vi "set decimali misure.vi"(6 "medie":i32[](array[numeric]), 8 "Abilita medie":bool, 9 "Filtro":bool[](array[boolean]), 10 "MISURE in":string[](array[string]), 11 "decimali":i32[](array[numeric])) -> (3 "MISURE out":string[](array[string]))   [LabVIEW 2019]
uses:
  <vilib>/ptbypt/NI_PtbyPt.lvlib
panel:
  out "Array":i32[](array[numeric])
  out "Numeric":i32
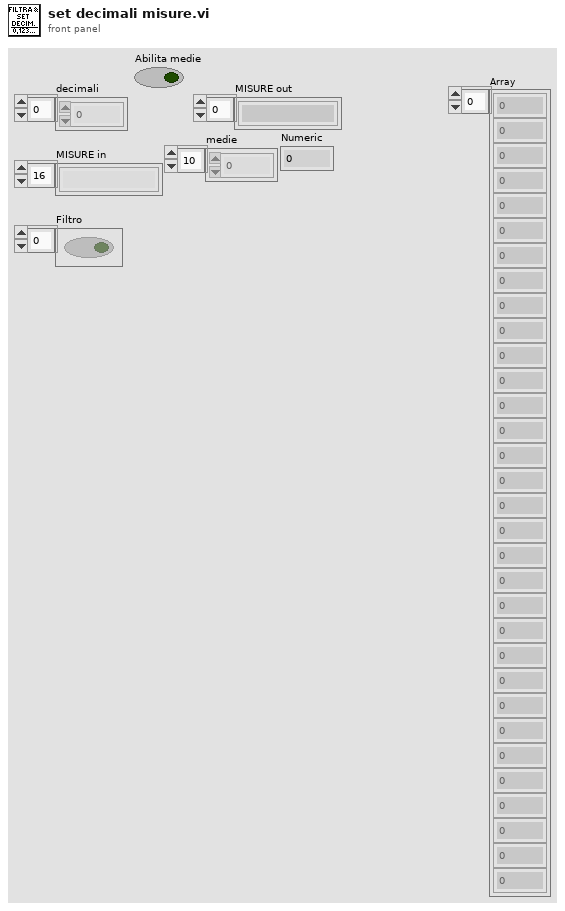
[diagram p1: front panel]
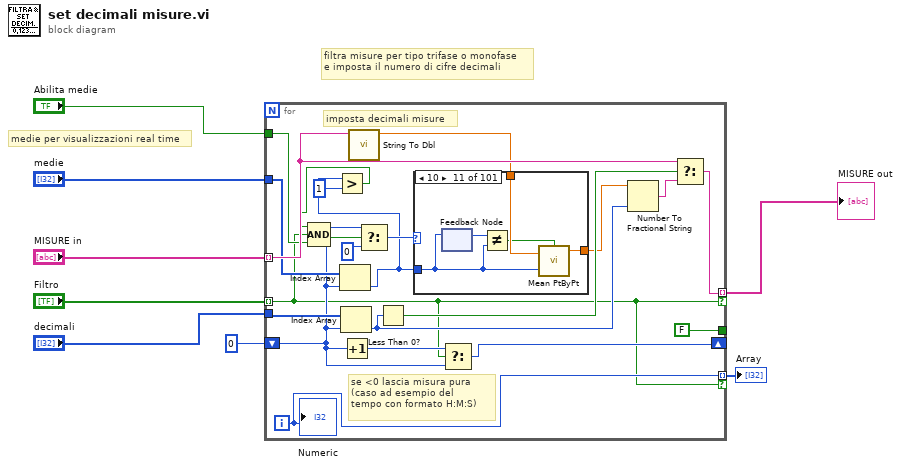
[diagram p0: block diagram]
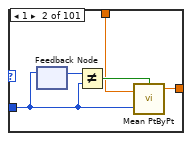
[diagram p3: hidden frame]
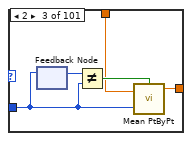
[diagram p4: hidden frame]
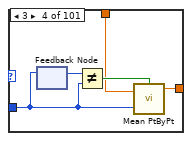
[diagram p5: hidden frame]
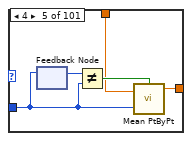
[diagram p6: hidden frame]
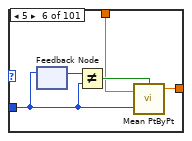
[diagram p7: hidden frame]
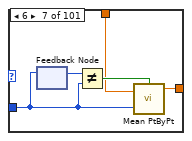
[diagram p8: hidden frame]
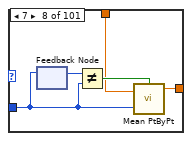
[diagram p9: hidden frame]
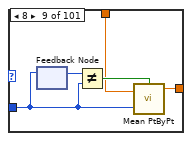
[diagram p10: hidden frame]
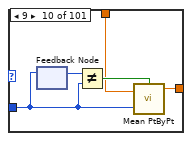
[diagram p11: hidden frame]
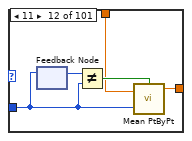
[diagram p12: hidden frame]
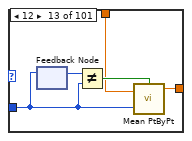
[diagram p13: hidden frame]
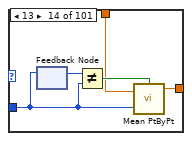
[diagram p14: hidden frame]
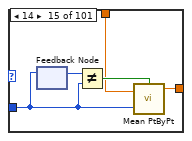
[diagram p15: hidden frame]
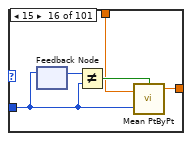
[diagram p16: hidden frame]
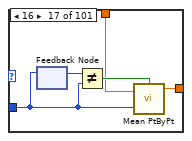
[diagram p17: hidden frame]
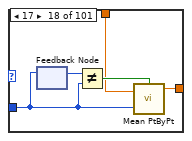
[diagram p18: hidden frame]
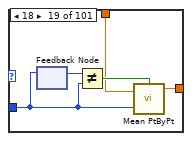
[diagram p19: hidden frame]
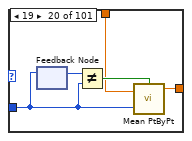
[diagram p20: hidden frame]
diagram:
  # "medie per visualizzazioni real time"
  # "filtra misure per tipo trifase o monofase\ne imposta il numero di cifre decimali"
  n1 = for {
    tunnel: "MISURE in" -> [w23] mode=indexing
    tunnel: [w24] -> w8 mode=indexing if=w9
    tunnel: [FALSE] -> _
    shift-right: [w29] -> _
    shift-left: 0 -> [w16]
    tunnel: "Filtro" -> [w9] mode=indexing
    tunnel: "decimali" -> [w27]
    tunnel: "medie" -> [w17]
    tunnel: "Abilita medie" -> [w15]
    tunnel: [w10] -> w1 mode=indexing if=w9
    i -> [w10]
    # "se <0 lascia misura pura\n(caso ad esempio del\ntempo con formato H:M:S)"
    # "imposta decimali misure"
    n2 = Index Array(array=w17, index=w16) -> (element=w13:i32)
    n3 = Greater?(x=w13, y=1) -> (0:w11:bool)
    n4 = Compound Arithmetic op=AND(w11, w9, w15) -> (w14:bool)
    n5 = Index Array(array=w27, index=w16) -> (element=w26:i32)
    n6 = Increment(x=w16) -> (x+1=w28:i32)
    n7 = call "String To Dbl.vi"("String"=w23) -> ("Numeric"=w20:dbl)  [unwired: 10 in]
    n8 = Select(t=w16, s=w14, f=0) -> (s? t:f=w19:i32)
    n9 = Less Than 0?(x=w26) -> (x < 0?=w22:bool)
    n10 = case shown="10" w19 {
      tunnel: w13 -> [_ w32 w37 w42 w47 w52 w57 w62 w67 w72 w78 w82 w87 w92 w97 w102 w107 w112 w117 w122 w127 w132 w137 w142 w147 w152 w157 w162 w167 w172 w177 w182 w187 w192 w197 w202 w207 w212 w217 w222 w227 w232 w237 w242 w247 w252 w257 w262 w267 w272 w277 w282 w287 w292 w297 w302 w307 w312 w317 w322 w327 w332 w337 w342 w347 w352 w357 w362 w367 w372 w377 w382 w387 w392 w397 w402 w407 w412 w417 w422 w427 w432 w437 w442 w447 w452 w457 w462 w467 w472 w477 w482 w487 w492 w497 w502 w507 w512 w517 w522 w527]
      tunnel: [w31 w34 w39 w44 w49 w54 w59 w64 w69 w74 w80 w84 w89 w94 w99 w104 w109 w114 w119 w124 w129 w134 w139 w144 w149 w154 w159 w164 w169 w174 w179 w184 w189 w194 w199 w204 w209 w214 w219 w224 w229 w234 w239 w244 w249 w254 w259 w264 w269 w274 w279 w284 w289 w294 w299 w304 w309 w314 w319 w324 w329 w334 w339 w344 w349 w354 w359 w364 w369 w374 w379 w384 w389 w394 w399 w404 w409 w414 w419 w424 w429 w434 w439 w444 w449 w454 w459 w464 w469 w474 w479 w484 w489 w494 w499 w504 w509 w514 w519 w524 w529] -> w21
      tunnel: w20 -> [w31 w33 w38 w43 w48 w53 w58 w63 w68 w73 w79 w83 w88 w93 w98 w103 w108 w113 w118 w123 w128 w133 w138 w143 w148 w153 w158 w163 w168 w173 w178 w183 w188 w193 w198 w203 w208 w213 w218 w223 w228 w233 w238 w243 w248 w253 w258 w263 w268 w273 w278 w283 w288 w293 w298 w303 w308 w313 w318 w323 w328 w333 w338 w343 w348 w353 w358 w363 w368 w373 w378 w383 w388 w393 w398 w403 w408 w413 w418 w423 w428 w433 w438 w443 w448 w453 w458 w463 w468 w473 w478 w483 w488 w493 w498 w503 w508 w513 w518 w523 w528]
      frame 0, Default {
      }
      frame 1 {
        n11 = feedback #1() -> (w35:i32)  [unwired: 1 in]
        n12 = feedback-in #1(w32) -> ()
        n13 = Not Equal?(x=w35, y=w32) -> (x != y?=w36:bool)
        n14 = call <vilib>:"Mean PtByPt.vi"("x"=w33, "sample length"=w32, "initialize"=w36) -> ("mean"=w34:dbl)  [unwired: 1 in, 1 out]
      }
      frame 2 {
        n15 = feedback #2() -> (w40:i32)  [unwired: 1 in]
        n16 = feedback-in #2(w37) -> ()
        n17 = Not Equal?(x=w40, y=w37) -> (x != y?=w41:bool)
        n18 = call <vilib>:"Mean PtByPt.vi"("x"=w38, "sample length"=w37, "initialize"=w41) -> ("mean"=w39:dbl)  [unwired: 1 in, 1 out]
      }
      frame 3 {
        n19 = feedback #3() -> (w45:i32)  [unwired: 1 in]
        n20 = feedback-in #3(w42) -> ()
        n21 = Not Equal?(x=w45, y=w42) -> (x != y?=w46:bool)
        n22 = call <vilib>:"Mean PtByPt.vi"("x"=w43, "sample length"=w42, "initialize"=w46) -> ("mean"=w44:dbl)  [unwired: 1 in, 1 out]
      }
      frame 4 {
        n23 = feedback #4() -> (w50:i32)  [unwired: 1 in]
        n24 = feedback-in #4(w47) -> ()
        n25 = Not Equal?(x=w50, y=w47) -> (x != y?=w51:bool)
        n26 = call <vilib>:"Mean PtByPt.vi"("x"=w48, "sample length"=w47, "initialize"=w51) -> ("mean"=w49:dbl)  [unwired: 1 in, 1 out]
      }
      frame 5 {
        n27 = feedback #5() -> (w55:i32)  [unwired: 1 in]
        n28 = feedback-in #5(w52) -> ()
        n29 = Not Equal?(x=w55, y=w52) -> (x != y?=w56:bool)
        n30 = call <vilib>:"Mean PtByPt.vi"("x"=w53, "sample length"=w52, "initialize"=w56) -> ("mean"=w54:dbl)  [unwired: 1 in, 1 out]
      }
      frame 6 {
        n31 = feedback #6() -> (w60:i32)  [unwired: 1 in]
        n32 = feedback-in #6(w57) -> ()
        n33 = Not Equal?(x=w60, y=w57) -> (x != y?=w61:bool)
        n34 = call <vilib>:"Mean PtByPt.vi"("x"=w58, "sample length"=w57, "initialize"=w61) -> ("mean"=w59:dbl)  [unwired: 1 in, 1 out]
      }
      frame 7 {
        n35 = feedback #7() -> (w65:i32)  [unwired: 1 in]
        n36 = feedback-in #7(w62) -> ()
        n37 = Not Equal?(x=w65, y=w62) -> (x != y?=w66:bool)
        n38 = call <vilib>:"Mean PtByPt.vi"("x"=w63, "sample length"=w62, "initialize"=w66) -> ("mean"=w64:dbl)  [unwired: 1 in, 1 out]
      }
      frame 8 {
        n39 = feedback #8() -> (w70:i32)  [unwired: 1 in]
        n40 = feedback-in #8(w67) -> ()
        n41 = Not Equal?(x=w70, y=w67) -> (x != y?=w71:bool)
        n42 = call <vilib>:"Mean PtByPt.vi"("x"=w68, "sample length"=w67, "initialize"=w71) -> ("mean"=w69:dbl)  [unwired: 1 in, 1 out]
      }
      frame 9 {
        n43 = feedback #9() -> (w75:i32)  [unwired: 1 in]
        n44 = feedback-in #9(w72) -> ()
        n45 = Not Equal?(x=w75, y=w72) -> (x != y?=w76:bool)
        n46 = call <vilib>:"Mean PtByPt.vi"("x"=w73, "sample length"=w72, "initialize"=w76) -> ("mean"=w74:dbl)  [unwired: 1 in, 1 out]
      }
      frame 10 {
        n47 = feedback #10() -> (w81:i32)  [unwired: 1 in]
        n48 = feedback-in #10(w78) -> ()
        n49 = Not Equal?(x=w81, y=w78) -> (x != y?=w77:bool)
        n50 = call <vilib>:"Mean PtByPt.vi"("x"=w79, "sample length"=w78, "initialize"=w77) -> ("mean"=w80:dbl)  [unwired: 1 in, 1 out]
      }
      frame 11 {
        n51 = feedback #11() -> (w85:i32)  [unwired: 1 in]
        n52 = feedback-in #11(w82) -> ()
        n53 = Not Equal?(x=w85, y=w82) -> (x != y?=w86:bool)
        n54 = call <vilib>:"Mean PtByPt.vi"("x"=w83, "sample length"=w82, "initialize"=w86) -> ("mean"=w84:dbl)  [unwired: 1 in, 1 out]
      }
      frame 12 {
        n55 = feedback #12() -> (w90:i32)  [unwired: 1 in]
        n56 = feedback-in #12(w87) -> ()
        n57 = Not Equal?(x=w90, y=w87) -> (x != y?=w91:bool)
        n58 = call <vilib>:"Mean PtByPt.vi"("x"=w88, "sample length"=w87, "initialize"=w91) -> ("mean"=w89:dbl)  [unwired: 1 in, 1 out]
      }
      frame 13 {
        n59 = feedback #13() -> (w95:i32)  [unwired: 1 in]
        n60 = feedback-in #13(w92) -> ()
        n61 = Not Equal?(x=w95, y=w92) -> (x != y?=w96:bool)
        n62 = call <vilib>:"Mean PtByPt.vi"("x"=w93, "sample length"=w92, "initialize"=w96) -> ("mean"=w94:dbl)  [unwired: 1 in, 1 out]
      }
      frame 14 {
        n63 = feedback #14() -> (w100:i32)  [unwired: 1 in]
        n64 = feedback-in #14(w97) -> ()
        n65 = Not Equal?(x=w100, y=w97) -> (x != y?=w101:bool)
        n66 = call <vilib>:"Mean PtByPt.vi"("x"=w98, "sample length"=w97, "initialize"=w101) -> ("mean"=w99:dbl)  [unwired: 1 in, 1 out]
      }
      frame 15 {
        n67 = feedback #15() -> (w105:i32)  [unwired: 1 in]
        n68 = feedback-in #15(w102) -> ()
        n69 = Not Equal?(x=w105, y=w102) -> (x != y?=w106:bool)
        n70 = call <vilib>:"Mean PtByPt.vi"("x"=w103, "sample length"=w102, "initialize"=w106) -> ("mean"=w104:dbl)  [unwired: 1 in, 1 out]
      }
      frame 16 {
        n71 = feedback #16() -> (w110:i32)  [unwired: 1 in]
        n72 = feedback-in #16(w107) -> ()
        n73 = Not Equal?(x=w110, y=w107) -> (x != y?=w111:bool)
        n74 = call <vilib>:"Mean PtByPt.vi"("x"=w108, "sample length"=w107, "initialize"=w111) -> ("mean"=w109:dbl)  [unwired: 1 in, 1 out]
      }
      frame 17 {
        n75 = feedback #17() -> (w115:i32)  [unwired: 1 in]
        n76 = feedback-in #17(w112) -> ()
        n77 = Not Equal?(x=w115, y=w112) -> (x != y?=w116:bool)
        n78 = call <vilib>:"Mean PtByPt.vi"("x"=w113, "sample length"=w112, "initialize"=w116) -> ("mean"=w114:dbl)  [unwired: 1 in, 1 out]
      }
      frame 18 {
        n79 = feedback #18() -> (w120:i32)  [unwired: 1 in]
        n80 = feedback-in #18(w117) -> ()
        n81 = Not Equal?(x=w120, y=w117) -> (x != y?=w121:bool)
        n82 = call <vilib>:"Mean PtByPt.vi"("x"=w118, "sample length"=w117, "initialize"=w121) -> ("mean"=w119:dbl)  [unwired: 1 in, 1 out]
      }
      frame 19 {
        n83 = feedback #19() -> (w125:i32)  [unwired: 1 in]
        n84 = feedback-in #19(w122) -> ()
        n85 = Not Equal?(x=w125, y=w122) -> (x != y?=w126:bool)
        n86 = call <vilib>:"Mean PtByPt.vi"("x"=w123, "sample length"=w122, "initialize"=w126) -> ("mean"=w124:dbl)  [unwired: 1 in, 1 out]
      }
      frame 20 {
        n87 = feedback #20() -> (w130:i32)  [unwired: 1 in]
        n88 = feedback-in #20(w127) -> ()
        n89 = Not Equal?(x=w130, y=w127) -> (x != y?=w131:bool)
        n90 = call <vilib>:"Mean PtByPt.vi"("x"=w128, "sample length"=w127, "initialize"=w131) -> ("mean"=w129:dbl)  [unwired: 1 in, 1 out]
      }
      frame 21 {
        n91 = feedback #21() -> (w135:i32)  [unwired: 1 in]
        n92 = feedback-in #21(w132) -> ()
        n93 = Not Equal?(x=w135, y=w132) -> (x != y?=w136:bool)
        n94 = call <vilib>:"Mean PtByPt.vi"("x"=w133, "sample length"=w132, "initialize"=w136) -> ("mean"=w134:dbl)  [unwired: 1 in, 1 out]
      }
      frame 22 {
        n95 = feedback #22() -> (w140:i32)  [unwired: 1 in]
        n96 = feedback-in #22(w137) -> ()
        n97 = Not Equal?(x=w140, y=w137) -> (x != y?=w141:bool)
        n98 = call <vilib>:"Mean PtByPt.vi"("x"=w138, "sample length"=w137, "initialize"=w141) -> ("mean"=w139:dbl)  [unwired: 1 in, 1 out]
      }
      frame 23 {
        n99 = feedback #23() -> (w145:i32)  [unwired: 1 in]
        n100 = feedback-in #23(w142) -> ()
        n101 = Not Equal?(x=w145, y=w142) -> (x != y?=w146:bool)
        n102 = call <vilib>:"Mean PtByPt.vi"("x"=w143, "sample length"=w142, "initialize"=w146) -> ("mean"=w144:dbl)  [unwired: 1 in, 1 out]
      }
      frame 24 {
        n103 = feedback #24() -> (w150:i32)  [unwired: 1 in]
        n104 = feedback-in #24(w147) -> ()
        n105 = Not Equal?(x=w150, y=w147) -> (x != y?=w151:bool)
        n106 = call <vilib>:"Mean PtByPt.vi"("x"=w148, "sample length"=w147, "initialize"=w151) -> ("mean"=w149:dbl)  [unwired: 1 in, 1 out]
      }
      frame 25 {
        n107 = feedback #25() -> (w155:i32)  [unwired: 1 in]
        n108 = feedback-in #25(w152) -> ()
        n109 = Not Equal?(x=w155, y=w152) -> (x != y?=w156:bool)
        n110 = call <vilib>:"Mean PtByPt.vi"("x"=w153, "sample length"=w152, "initialize"=w156) -> ("mean"=w154:dbl)  [unwired: 1 in, 1 out]
      }
      frame 26 {
        n111 = feedback #26() -> (w160:i32)  [unwired: 1 in]
        n112 = feedback-in #26(w157) -> ()
        n113 = Not Equal?(x=w160, y=w157) -> (x != y?=w161:bool)
        n114 = call <vilib>:"Mean PtByPt.vi"("x"=w158, "sample length"=w157, "initialize"=w161) -> ("mean"=w159:dbl)  [unwired: 1 in, 1 out]
      }
      frame 27 {
        n115 = feedback #27() -> (w165:i32)  [unwired: 1 in]
        n116 = feedback-in #27(w162) -> ()
        n117 = Not Equal?(x=w165, y=w162) -> (x != y?=w166:bool)
        n118 = call <vilib>:"Mean PtByPt.vi"("x"=w163, "sample length"=w162, "initialize"=w166) -> ("mean"=w164:dbl)  [unwired: 1 in, 1 out]
      }
      frame 28 {
        n119 = feedback #28() -> (w170:i32)  [unwired: 1 in]
        n120 = feedback-in #28(w167) -> ()
        n121 = Not Equal?(x=w170, y=w167) -> (x != y?=w171:bool)
        n122 = call <vilib>:"Mean PtByPt.vi"("x"=w168, "sample length"=w167, "initialize"=w171) -> ("mean"=w169:dbl)  [unwired: 1 in, 1 out]
      }
      frame 29 {
        n123 = feedback #29() -> (w175:i32)  [unwired: 1 in]
        n124 = feedback-in #29(w172) -> ()
        n125 = Not Equal?(x=w175, y=w172) -> (x != y?=w176:bool)
        n126 = call <vilib>:"Mean PtByPt.vi"("x"=w173, "sample length"=w172, "initialize"=w176) -> ("mean"=w174:dbl)  [unwired: 1 in, 1 out]
      }
      frame 30 {
        n127 = feedback #30() -> (w180:i32)  [unwired: 1 in]
        n128 = feedback-in #30(w177) -> ()
        n129 = Not Equal?(x=w180, y=w177) -> (x != y?=w181:bool)
        n130 = call <vilib>:"Mean PtByPt.vi"("x"=w178, "sample length"=w177, "initialize"=w181) -> ("mean"=w179:dbl)  [unwired: 1 in, 1 out]
      }
      frame 31 {
        n131 = feedback #31() -> (w185:i32)  [unwired: 1 in]
        n132 = feedback-in #31(w182) -> ()
        n133 = Not Equal?(x=w185, y=w182) -> (x != y?=w186:bool)
        n134 = call <vilib>:"Mean PtByPt.vi"("x"=w183, "sample length"=w182, "initialize"=w186) -> ("mean"=w184:dbl)  [unwired: 1 in, 1 out]
      }
      frame 32 {
        n135 = feedback #32() -> (w190:i32)  [unwired: 1 in]
        n136 = feedback-in #32(w187) -> ()
        n137 = Not Equal?(x=w190, y=w187) -> (x != y?=w191:bool)
        n138 = call <vilib>:"Mean PtByPt.vi"("x"=w188, "sample length"=w187, "initialize"=w191) -> ("mean"=w189:dbl)  [unwired: 1 in, 1 out]
      }
      frame 33 {
        n139 = feedback #33() -> (w195:i32)  [unwired: 1 in]
        n140 = feedback-in #33(w192) -> ()
        n141 = Not Equal?(x=w195, y=w192) -> (x != y?=w196:bool)
        n142 = call <vilib>:"Mean PtByPt.vi"("x"=w193, "sample length"=w192, "initialize"=w196) -> ("mean"=w194:dbl)  [unwired: 1 in, 1 out]
      }
      frame 34 {
        n143 = feedback #34() -> (w200:i32)  [unwired: 1 in]
        n144 = feedback-in #34(w197) -> ()
        n145 = Not Equal?(x=w200, y=w197) -> (x != y?=w201:bool)
        n146 = call <vilib>:"Mean PtByPt.vi"("x"=w198, "sample length"=w197, "initialize"=w201) -> ("mean"=w199:dbl)  [unwired: 1 in, 1 out]
      }
      frame 35 {
        n147 = feedback #35() -> (w205:i32)  [unwired: 1 in]
        n148 = feedback-in #35(w202) -> ()
        n149 = Not Equal?(x=w205, y=w202) -> (x != y?=w206:bool)
        n150 = call <vilib>:"Mean PtByPt.vi"("x"=w203, "sample length"=w202, "initialize"=w206) -> ("mean"=w204:dbl)  [unwired: 1 in, 1 out]
      }
      frame 36 {
        n151 = feedback #36() -> (w210:i32)  [unwired: 1 in]
        n152 = feedback-in #36(w207) -> ()
        n153 = Not Equal?(x=w210, y=w207) -> (x != y?=w211:bool)
        n154 = call <vilib>:"Mean PtByPt.vi"("x"=w208, "sample length"=w207, "initialize"=w211) -> ("mean"=w209:dbl)  [unwired: 1 in, 1 out]
      }
      frame 37 {
        n155 = feedback #37() -> (w215:i32)  [unwired: 1 in]
        n156 = feedback-in #37(w212) -> ()
        n157 = Not Equal?(x=w215, y=w212) -> (x != y?=w216:bool)
        n158 = call <vilib>:"Mean PtByPt.vi"("x"=w213, "sample length"=w212, "initialize"=w216) -> ("mean"=w214:dbl)  [unwired: 1 in, 1 out]
      }
      frame 38 {
        n159 = feedback #38() -> (w220:i32)  [unwired: 1 in]
        n160 = feedback-in #38(w217) -> ()
        n161 = Not Equal?(x=w220, y=w217) -> (x != y?=w221:bool)
        n162 = call <vilib>:"Mean PtByPt.vi"("x"=w218, "sample length"=w217, "initialize"=w221) -> ("mean"=w219:dbl)  [unwired: 1 in, 1 out]
      }
      frame 39 {
        n163 = feedback #39() -> (w225:i32)  [unwired: 1 in]
        n164 = feedback-in #39(w222) -> ()
        n165 = Not Equal?(x=w225, y=w222) -> (x != y?=w226:bool)
        n166 = call <vilib>:"Mean PtByPt.vi"("x"=w223, "sample length"=w222, "initialize"=w226) -> ("mean"=w224:dbl)  [unwired: 1 in, 1 out]
      }
      frame 40 {
        n167 = feedback #40() -> (w230:i32)  [unwired: 1 in]
        n168 = feedback-in #40(w227) -> ()
        n169 = Not Equal?(x=w230, y=w227) -> (x != y?=w231:bool)
        n170 = call <vilib>:"Mean PtByPt.vi"("x"=w228, "sample length"=w227, "initialize"=w231) -> ("mean"=w229:dbl)  [unwired: 1 in, 1 out]
      }
      frame 41 {
        n171 = feedback #41() -> (w235:i32)  [unwired: 1 in]
        n172 = feedback-in #41(w232) -> ()
        n173 = Not Equal?(x=w235, y=w232) -> (x != y?=w236:bool)
        n174 = call <vilib>:"Mean PtByPt.vi"("x"=w233, "sample length"=w232, "initialize"=w236) -> ("mean"=w234:dbl)  [unwired: 1 in, 1 out]
      }
      frame 42 {
        n175 = feedback #42() -> (w240:i32)  [unwired: 1 in]
        n176 = feedback-in #42(w237) -> ()
        n177 = Not Equal?(x=w240, y=w237) -> (x != y?=w241:bool)
        n178 = call <vilib>:"Mean PtByPt.vi"("x"=w238, "sample length"=w237, "initialize"=w241) -> ("mean"=w239:dbl)  [unwired: 1 in, 1 out]
      }
      frame 43 {
        n179 = feedback #43() -> (w245:i32)  [unwired: 1 in]
        n180 = feedback-in #43(w242) -> ()
        n181 = Not Equal?(x=w245, y=w242) -> (x != y?=w246:bool)
        n182 = call <vilib>:"Mean PtByPt.vi"("x"=w243, "sample length"=w242, "initialize"=w246) -> ("mean"=w244:dbl)  [unwired: 1 in, 1 out]
      }
      frame 44 {
        n183 = feedback #44() -> (w250:i32)  [unwired: 1 in]
        n184 = feedback-in #44(w247) -> ()
        n185 = Not Equal?(x=w250, y=w247) -> (x != y?=w251:bool)
        n186 = call <vilib>:"Mean PtByPt.vi"("x"=w248, "sample length"=w247, "initialize"=w251) -> ("mean"=w249:dbl)  [unwired: 1 in, 1 out]
      }
      frame 45 {
        n187 = feedback #45() -> (w255:i32)  [unwired: 1 in]
        n188 = feedback-in #45(w252) -> ()
        n189 = Not Equal?(x=w255, y=w252) -> (x != y?=w256:bool)
        n190 = call <vilib>:"Mean PtByPt.vi"("x"=w253, "sample length"=w252, "initialize"=w256) -> ("mean"=w254:dbl)  [unwired: 1 in, 1 out]
      }
      frame 46 {
        n191 = feedback #46() -> (w260:i32)  [unwired: 1 in]
        n192 = feedback-in #46(w257) -> ()
        n193 = Not Equal?(x=w260, y=w257) -> (x != y?=w261:bool)
        n194 = call <vilib>:"Mean PtByPt.vi"("x"=w258, "sample length"=w257, "initialize"=w261) -> ("mean"=w259:dbl)  [unwired: 1 in, 1 out]
      }
      frame 47 {
        n195 = feedback #47() -> (w265:i32)  [unwired: 1 in]
        n196 = feedback-in #47(w262) -> ()
        n197 = Not Equal?(x=w265, y=w262) -> (x != y?=w266:bool)
        n198 = call <vilib>:"Mean PtByPt.vi"("x"=w263, "sample length"=w262, "initialize"=w266) -> ("mean"=w264:dbl)  [unwired: 1 in, 1 out]
      }
      frame 48 {
        n199 = feedback #48() -> (w270:i32)  [unwired: 1 in]
        n200 = feedback-in #48(w267) -> ()
        n201 = Not Equal?(x=w270, y=w267) -> (x != y?=w271:bool)
        n202 = call <vilib>:"Mean PtByPt.vi"("x"=w268, "sample length"=w267, "initialize"=w271) -> ("mean"=w269:dbl)  [unwired: 1 in, 1 out]
      }
      frame 49 {
        n203 = feedback #49() -> (w275:i32)  [unwired: 1 in]
        n204 = feedback-in #49(w272) -> ()
        n205 = Not Equal?(x=w275, y=w272) -> (x != y?=w276:bool)
        n206 = call <vilib>:"Mean PtByPt.vi"("x"=w273, "sample length"=w272, "initialize"=w276) -> ("mean"=w274:dbl)  [unwired: 1 in, 1 out]
      }
      frame 50 {
        n207 = feedback #50() -> (w280:i32)  [unwired: 1 in]
        n208 = feedback-in #50(w277) -> ()
        n209 = Not Equal?(x=w280, y=w277) -> (x != y?=w281:bool)
        n210 = call <vilib>:"Mean PtByPt.vi"("x"=w278, "sample length"=w277, "initialize"=w281) -> ("mean"=w279:dbl)  [unwired: 1 in, 1 out]
      }
      frame 51 {
        n211 = feedback #51() -> (w285:i32)  [unwired: 1 in]
        n212 = feedback-in #51(w282) -> ()
        n213 = Not Equal?(x=w285, y=w282) -> (x != y?=w286:bool)
        n214 = call <vilib>:"Mean PtByPt.vi"("x"=w283, "sample length"=w282, "initialize"=w286) -> ("mean"=w284:dbl)  [unwired: 1 in, 1 out]
      }
      frame 52 {
        n215 = feedback #52() -> (w290:i32)  [unwired: 1 in]
        n216 = feedback-in #52(w287) -> ()
        n217 = Not Equal?(x=w290, y=w287) -> (x != y?=w291:bool)
        n218 = call <vilib>:"Mean PtByPt.vi"("x"=w288, "sample length"=w287, "initialize"=w291) -> ("mean"=w289:dbl)  [unwired: 1 in, 1 out]
      }
      frame 53 {
        n219 = feedback #53() -> (w295:i32)  [unwired: 1 in]
        n220 = feedback-in #53(w292) -> ()
        n221 = Not Equal?(x=w295, y=w292) -> (x != y?=w296:bool)
        n222 = call <vilib>:"Mean PtByPt.vi"("x"=w293, "sample length"=w292, "initialize"=w296) -> ("mean"=w294:dbl)  [unwired: 1 in, 1 out]
      }
      frame 54 {
        n223 = feedback #54() -> (w300:i32)  [unwired: 1 in]
        n224 = feedback-in #54(w297) -> ()
        n225 = Not Equal?(x=w300, y=w297) -> (x != y?=w301:bool)
        n226 = call <vilib>:"Mean PtByPt.vi"("x"=w298, "sample length"=w297, "initialize"=w301) -> ("mean"=w299:dbl)  [unwired: 1 in, 1 out]
      }
      frame 55 {
        n227 = feedback #55() -> (w305:i32)  [unwired: 1 in]
        n228 = feedback-in #55(w302) -> ()
        n229 = Not Equal?(x=w305, y=w302) -> (x != y?=w306:bool)
        n230 = call <vilib>:"Mean PtByPt.vi"("x"=w303, "sample length"=w302, "initialize"=w306) -> ("mean"=w304:dbl)  [unwired: 1 in, 1 out]
      }
      frame 56 {
        n231 = feedback #56() -> (w310:i32)  [unwired: 1 in]
        n232 = feedback-in #56(w307) -> ()
        n233 = Not Equal?(x=w310, y=w307) -> (x != y?=w311:bool)
        n234 = call <vilib>:"Mean PtByPt.vi"("x"=w308, "sample length"=w307, "initialize"=w311) -> ("mean"=w309:dbl)  [unwired: 1 in, 1 out]
      }
      frame 57 {
        n235 = feedback #57() -> (w315:i32)  [unwired: 1 in]
        n236 = feedback-in #57(w312) -> ()
        n237 = Not Equal?(x=w315, y=w312) -> (x != y?=w316:bool)
        n238 = call <vilib>:"Mean PtByPt.vi"("x"=w313, "sample length"=w312, "initialize"=w316) -> ("mean"=w314:dbl)  [unwired: 1 in, 1 out]
      }
      frame 58 {
        n239 = feedback #58() -> (w320:i32)  [unwired: 1 in]
        n240 = feedback-in #58(w317) -> ()
        n241 = Not Equal?(x=w320, y=w317) -> (x != y?=w321:bool)
        n242 = call <vilib>:"Mean PtByPt.vi"("x"=w318, "sample length"=w317, "initialize"=w321) -> ("mean"=w319:dbl)  [unwired: 1 in, 1 out]
      }
      frame 59 {
        n243 = feedback #59() -> (w325:i32)  [unwired: 1 in]
        n244 = feedback-in #59(w322) -> ()
        n245 = Not Equal?(x=w325, y=w322) -> (x != y?=w326:bool)
        n246 = call <vilib>:"Mean PtByPt.vi"("x"=w323, "sample length"=w322, "initialize"=w326) -> ("mean"=w324:dbl)  [unwired: 1 in, 1 out]
      }
      frame 60 {
        n247 = feedback #60() -> (w330:i32)  [unwired: 1 in]
        n248 = feedback-in #60(w327) -> ()
        n249 = Not Equal?(x=w330, y=w327) -> (x != y?=w331:bool)
        n250 = call <vilib>:"Mean PtByPt.vi"("x"=w328, "sample length"=w327, "initialize"=w331) -> ("mean"=w329:dbl)  [unwired: 1 in, 1 out]
      }
      frame 61 {
        n251 = feedback #61() -> (w335:i32)  [unwired: 1 in]
        n252 = feedback-in #61(w332) -> ()
        n253 = Not Equal?(x=w335, y=w332) -> (x != y?=w336:bool)
        n254 = call <vilib>:"Mean PtByPt.vi"("x"=w333, "sample length"=w332, "initialize"=w336) -> ("mean"=w334:dbl)  [unwired: 1 in, 1 out]
      }
      frame 62 {
        n255 = feedback #62() -> (w340:i32)  [unwired: 1 in]
        n256 = feedback-in #62(w337) -> ()
        n257 = Not Equal?(x=w340, y=w337) -> (x != y?=w341:bool)
        n258 = call <vilib>:"Mean PtByPt.vi"("x"=w338, "sample length"=w337, "initialize"=w341) -> ("mean"=w339:dbl)  [unwired: 1 in, 1 out]
      }
      frame 63 {
        n259 = feedback #63() -> (w345:i32)  [unwired: 1 in]
        n260 = feedback-in #63(w342) -> ()
        n261 = Not Equal?(x=w345, y=w342) -> (x != y?=w346:bool)
        n262 = call <vilib>:"Mean PtByPt.vi"("x"=w343, "sample length"=w342, "initialize"=w346) -> ("mean"=w344:dbl)  [unwired: 1 in, 1 out]
      }
      frame 64 {
        n263 = feedback #64() -> (w350:i32)  [unwired: 1 in]
        n264 = feedback-in #64(w347) -> ()
        n265 = Not Equal?(x=w350, y=w347) -> (x != y?=w351:bool)
        n266 = call <vilib>:"Mean PtByPt.vi"("x"=w348, "sample length"=w347, "initialize"=w351) -> ("mean"=w349:dbl)  [unwired: 1 in, 1 out]
      }
      frame 65 {
        n267 = feedback #65() -> (w355:i32)  [unwired: 1 in]
        n268 = feedback-in #65(w352) -> ()
        n269 = Not Equal?(x=w355, y=w352) -> (x != y?=w356:bool)
        n270 = call <vilib>:"Mean PtByPt.vi"("x"=w353, "sample length"=w352, "initialize"=w356) -> ("mean"=w354:dbl)  [unwired: 1 in, 1 out]
      }
      frame 66 {
        n271 = feedback #66() -> (w360:i32)  [unwired: 1 in]
        n272 = feedback-in #66(w357) -> ()
        n273 = Not Equal?(x=w360, y=w357) -> (x != y?=w361:bool)
        n274 = call <vilib>:"Mean PtByPt.vi"("x"=w358, "sample length"=w357, "initialize"=w361) -> ("mean"=w359:dbl)  [unwired: 1 in, 1 out]
      }
      frame 67 {
        n275 = feedback #67() -> (w365:i32)  [unwired: 1 in]
        n276 = feedback-in #67(w362) -> ()
        n277 = Not Equal?(x=w365, y=w362) -> (x != y?=w366:bool)
        n278 = call <vilib>:"Mean PtByPt.vi"("x"=w363, "sample length"=w362, "initialize"=w366) -> ("mean"=w364:dbl)  [unwired: 1 in, 1 out]
      }
      frame 68 {
        n279 = feedback #68() -> (w370:i32)  [unwired: 1 in]
        n280 = feedback-in #68(w367) -> ()
        n281 = Not Equal?(x=w370, y=w367) -> (x != y?=w371:bool)
        n282 = call <vilib>:"Mean PtByPt.vi"("x"=w368, "sample length"=w367, "initialize"=w371) -> ("mean"=w369:dbl)  [unwired: 1 in, 1 out]
      }
      frame 69 {
        n283 = feedback #69() -> (w375:i32)  [unwired: 1 in]
        n284 = feedback-in #69(w372) -> ()
        n285 = Not Equal?(x=w375, y=w372) -> (x != y?=w376:bool)
        n286 = call <vilib>:"Mean PtByPt.vi"("x"=w373, "sample length"=w372, "initialize"=w376) -> ("mean"=w374:dbl)  [unwired: 1 in, 1 out]
      }
      frame 70 {
        n287 = feedback #70() -> (w380:i32)  [unwired: 1 in]
        n288 = feedback-in #70(w377) -> ()
        n289 = Not Equal?(x=w380, y=w377) -> (x != y?=w381:bool)
        n290 = call <vilib>:"Mean PtByPt.vi"("x"=w378, "sample length"=w377, "initialize"=w381) -> ("mean"=w379:dbl)  [unwired: 1 in, 1 out]
      }
      frame 71 {
        n291 = feedback #71() -> (w385:i32)  [unwired: 1 in]
        n292 = feedback-in #71(w382) -> ()
        n293 = Not Equal?(x=w385, y=w382) -> (x != y?=w386:bool)
        n294 = call <vilib>:"Mean PtByPt.vi"("x"=w383, "sample length"=w382, "initialize"=w386) -> ("mean"=w384:dbl)  [unwired: 1 in, 1 out]
      }
      frame 72 {
        n295 = feedback #72() -> (w390:i32)  [unwired: 1 in]
        n296 = feedback-in #72(w387) -> ()
        n297 = Not Equal?(x=w390, y=w387) -> (x != y?=w391:bool)
        n298 = call <vilib>:"Mean PtByPt.vi"("x"=w388, "sample length"=w387, "initialize"=w391) -> ("mean"=w389:dbl)  [unwired: 1 in, 1 out]
      }
      frame 73 {
        n299 = feedback #73() -> (w395:i32)  [unwired: 1 in]
        n300 = feedback-in #73(w392) -> ()
        n301 = Not Equal?(x=w395, y=w392) -> (x != y?=w396:bool)
        n302 = call <vilib>:"Mean PtByPt.vi"("x"=w393, "sample length"=w392, "initialize"=w396) -> ("mean"=w394:dbl)  [unwired: 1 in, 1 out]
      }
      frame 74 {
        n303 = feedback #74() -> (w400:i32)  [unwired: 1 in]
        n304 = feedback-in #74(w397) -> ()
        n305 = Not Equal?(x=w400, y=w397) -> (x != y?=w401:bool)
        n306 = call <vilib>:"Mean PtByPt.vi"("x"=w398, "sample length"=w397, "initialize"=w401) -> ("mean"=w399:dbl)  [unwired: 1 in, 1 out]
      }
      frame 75 {
        n307 = feedback #75() -> (w405:i32)  [unwired: 1 in]
        n308 = feedback-in #75(w402) -> ()
        n309 = Not Equal?(x=w405, y=w402) -> (x != y?=w406:bool)
        n310 = call <vilib>:"Mean PtByPt.vi"("x"=w403, "sample length"=w402, "initialize"=w406) -> ("mean"=w404:dbl)  [unwired: 1 in, 1 out]
      }
      frame 76 {
        n311 = feedback #76() -> (w410:i32)  [unwired: 1 in]
        n312 = feedback-in #76(w407) -> ()
        n313 = Not Equal?(x=w410, y=w407) -> (x != y?=w411:bool)
        n314 = call <vilib>:"Mean PtByPt.vi"("x"=w408, "sample length"=w407, "initialize"=w411) -> ("mean"=w409:dbl)  [unwired: 1 in, 1 out]
      }
      frame 77 {
        n315 = feedback #77() -> (w415:i32)  [unwired: 1 in]
        n316 = feedback-in #77(w412) -> ()
        n317 = Not Equal?(x=w415, y=w412) -> (x != y?=w416:bool)
        n318 = call <vilib>:"Mean PtByPt.vi"("x"=w413, "sample length"=w412, "initialize"=w416) -> ("mean"=w414:dbl)  [unwired: 1 in, 1 out]
      }
      frame 78 {
        n319 = feedback #78() -> (w420:i32)  [unwired: 1 in]
        n320 = feedback-in #78(w417) -> ()
        n321 = Not Equal?(x=w420, y=w417) -> (x != y?=w421:bool)
        n322 = call <vilib>:"Mean PtByPt.vi"("x"=w418, "sample length"=w417, "initialize"=w421) -> ("mean"=w419:dbl)  [unwired: 1 in, 1 out]
      }
      frame 79 {
        n323 = feedback #79() -> (w425:i32)  [unwired: 1 in]
        n324 = feedback-in #79(w422) -> ()
        n325 = Not Equal?(x=w425, y=w422) -> (x != y?=w426:bool)
        n326 = call <vilib>:"Mean PtByPt.vi"("x"=w423, "sample length"=w422, "initialize"=w426) -> ("mean"=w424:dbl)  [unwired: 1 in, 1 out]
      }
      frame 80 {
        n327 = feedback #80() -> (w430:i32)  [unwired: 1 in]
        n328 = feedback-in #80(w427) -> ()
        n329 = Not Equal?(x=w430, y=w427) -> (x != y?=w431:bool)
        n330 = call <vilib>:"Mean PtByPt.vi"("x"=w428, "sample length"=w427, "initialize"=w431) -> ("mean"=w429:dbl)  [unwired: 1 in, 1 out]
      }
      frame 81 {
        n331 = feedback #81() -> (w435:i32)  [unwired: 1 in]
        n332 = feedback-in #81(w432) -> ()
        n333 = Not Equal?(x=w435, y=w432) -> (x != y?=w436:bool)
        n334 = call <vilib>:"Mean PtByPt.vi"("x"=w433, "sample length"=w432, "initialize"=w436) -> ("mean"=w434:dbl)  [unwired: 1 in, 1 out]
      }
      frame 82 {
        n335 = feedback #82() -> (w440:i32)  [unwired: 1 in]
        n336 = feedback-in #82(w437) -> ()
        n337 = Not Equal?(x=w440, y=w437) -> (x != y?=w441:bool)
        n338 = call <vilib>:"Mean PtByPt.vi"("x"=w438, "sample length"=w437, "initialize"=w441) -> ("mean"=w439:dbl)  [unwired: 1 in, 1 out]
      }
      frame 83 {
        n339 = feedback #83() -> (w445:i32)  [unwired: 1 in]
        n340 = feedback-in #83(w442) -> ()
        n341 = Not Equal?(x=w445, y=w442) -> (x != y?=w446:bool)
        n342 = call <vilib>:"Mean PtByPt.vi"("x"=w443, "sample length"=w442, "initialize"=w446) -> ("mean"=w444:dbl)  [unwired: 1 in, 1 out]
      }
      frame 84 {
        n343 = feedback #84() -> (w450:i32)  [unwired: 1 in]
        n344 = feedback-in #84(w447) -> ()
        n345 = Not Equal?(x=w450, y=w447) -> (x != y?=w451:bool)
        n346 = call <vilib>:"Mean PtByPt.vi"("x"=w448, "sample length"=w447, "initialize"=w451) -> ("mean"=w449:dbl)  [unwired: 1 in, 1 out]
      }
      frame 85 {
        n347 = feedback #85() -> (w455:i32)  [unwired: 1 in]
        n348 = feedback-in #85(w452) -> ()
        n349 = Not Equal?(x=w455, y=w452) -> (x != y?=w456:bool)
        n350 = call <vilib>:"Mean PtByPt.vi"("x"=w453, "sample length"=w452, "initialize"=w456) -> ("mean"=w454:dbl)  [unwired: 1 in, 1 out]
      }
      frame 86 {
        n351 = feedback #86() -> (w460:i32)  [unwired: 1 in]
        n352 = feedback-in #86(w457) -> ()
        n353 = Not Equal?(x=w460, y=w457) -> (x != y?=w461:bool)
        n354 = call <vilib>:"Mean PtByPt.vi"("x"=w458, "sample length"=w457, "initialize"=w461) -> ("mean"=w459:dbl)  [unwired: 1 in, 1 out]
      }
      frame 87 {
        n355 = feedback #87() -> (w465:i32)  [unwired: 1 in]
        n356 = feedback-in #87(w462) -> ()
        n357 = Not Equal?(x=w465, y=w462) -> (x != y?=w466:bool)
        n358 = call <vilib>:"Mean PtByPt.vi"("x"=w463, "sample length"=w462, "initialize"=w466) -> ("mean"=w464:dbl)  [unwired: 1 in, 1 out]
      }
      frame 88 {
        n359 = feedback #88() -> (w470:i32)  [unwired: 1 in]
        n360 = feedback-in #88(w467) -> ()
        n361 = Not Equal?(x=w470, y=w467) -> (x != y?=w471:bool)
        n362 = call <vilib>:"Mean PtByPt.vi"("x"=w468, "sample length"=w467, "initialize"=w471) -> ("mean"=w469:dbl)  [unwired: 1 in, 1 out]
      }
      frame 89 {
        n363 = feedback #89() -> (w475:i32)  [unwired: 1 in]
        n364 = feedback-in #89(w472) -> ()
        n365 = Not Equal?(x=w475, y=w472) -> (x != y?=w476:bool)
        n366 = call <vilib>:"Mean PtByPt.vi"("x"=w473, "sample length"=w472, "initialize"=w476) -> ("mean"=w474:dbl)  [unwired: 1 in, 1 out]
      }
      frame 90 {
        n367 = feedback #90() -> (w480:i32)  [unwired: 1 in]
        n368 = feedback-in #90(w477) -> ()
        n369 = Not Equal?(x=w480, y=w477) -> (x != y?=w481:bool)
        n370 = call <vilib>:"Mean PtByPt.vi"("x"=w478, "sample length"=w477, "initialize"=w481) -> ("mean"=w479:dbl)  [unwired: 1 in, 1 out]
      }
      frame 91 {
        n371 = feedback #91() -> (w485:i32)  [unwired: 1 in]
        n372 = feedback-in #91(w482) -> ()
        n373 = Not Equal?(x=w485, y=w482) -> (x != y?=w486:bool)
        n374 = call <vilib>:"Mean PtByPt.vi"("x"=w483, "sample length"=w482, "initialize"=w486) -> ("mean"=w484:dbl)  [unwired: 1 in, 1 out]
      }
      frame 92 {
        n375 = feedback #92() -> (w490:i32)  [unwired: 1 in]
        n376 = feedback-in #92(w487) -> ()
        n377 = Not Equal?(x=w490, y=w487) -> (x != y?=w491:bool)
        n378 = call <vilib>:"Mean PtByPt.vi"("x"=w488, "sample length"=w487, "initialize"=w491) -> ("mean"=w489:dbl)  [unwired: 1 in, 1 out]
      }
      frame 93 {
        n379 = feedback #93() -> (w495:i32)  [unwired: 1 in]
        n380 = feedback-in #93(w492) -> ()
        n381 = Not Equal?(x=w495, y=w492) -> (x != y?=w496:bool)
        n382 = call <vilib>:"Mean PtByPt.vi"("x"=w493, "sample length"=w492, "initialize"=w496) -> ("mean"=w494:dbl)  [unwired: 1 in, 1 out]
      }
      frame 94 {
        n383 = feedback #94() -> (w500:i32)  [unwired: 1 in]
        n384 = feedback-in #94(w497) -> ()
        n385 = Not Equal?(x=w500, y=w497) -> (x != y?=w501:bool)
        n386 = call <vilib>:"Mean PtByPt.vi"("x"=w498, "sample length"=w497, "initialize"=w501) -> ("mean"=w499:dbl)  [unwired: 1 in, 1 out]
      }
      frame 95 {
        n387 = feedback #95() -> (w505:i32)  [unwired: 1 in]
        n388 = feedback-in #95(w502) -> ()
        n389 = Not Equal?(x=w505, y=w502) -> (x != y?=w506:bool)
        n390 = call <vilib>:"Mean PtByPt.vi"("x"=w503, "sample length"=w502, "initialize"=w506) -> ("mean"=w504:dbl)  [unwired: 1 in, 1 out]
      }
      frame 96 {
        n391 = feedback #96() -> (w510:i32)  [unwired: 1 in]
        n392 = feedback-in #96(w507) -> ()
        n393 = Not Equal?(x=w510, y=w507) -> (x != y?=w511:bool)
        n394 = call <vilib>:"Mean PtByPt.vi"("x"=w508, "sample length"=w507, "initialize"=w511) -> ("mean"=w509:dbl)  [unwired: 1 in, 1 out]
      }
      frame 97 {
        n395 = feedback #97() -> (w515:i32)  [unwired: 1 in]
        n396 = feedback-in #97(w512) -> ()
        n397 = Not Equal?(x=w515, y=w512) -> (x != y?=w516:bool)
        n398 = call <vilib>:"Mean PtByPt.vi"("x"=w513, "sample length"=w512, "initialize"=w516) -> ("mean"=w514:dbl)  [unwired: 1 in, 1 out]
      }
      frame 98 {
        n399 = feedback #98() -> (w520:i32)  [unwired: 1 in]
        n400 = feedback-in #98(w517) -> ()
        n401 = Not Equal?(x=w520, y=w517) -> (x != y?=w521:bool)
        n402 = call <vilib>:"Mean PtByPt.vi"("x"=w518, "sample length"=w517, "initialize"=w521) -> ("mean"=w519:dbl)  [unwired: 1 in, 1 out]
      }
      frame 99 {
        n403 = feedback #99() -> (w525:i32)  [unwired: 1 in]
        n404 = feedback-in #99(w522) -> ()
        n405 = Not Equal?(x=w525, y=w522) -> (x != y?=w526:bool)
        n406 = call <vilib>:"Mean PtByPt.vi"("x"=w523, "sample length"=w522, "initialize"=w526) -> ("mean"=w524:dbl)  [unwired: 1 in, 1 out]
      }
      frame 100 {
        n407 = feedback #100() -> (w530:i32)  [unwired: 1 in]
        n408 = feedback-in #100(w527) -> ()
        n409 = Not Equal?(x=w530, y=w527) -> (x != y?=w531:bool)
        n410 = call <vilib>:"Mean PtByPt.vi"("x"=w528, "sample length"=w527, "initialize"=w531) -> ("mean"=w529:dbl)  [unwired: 1 in, 1 out]
      }
    }
    n411 = Select(t=w28, s=w9, f=w16) -> (s? t:f=w29:i32)
    n412 = Number To Fractional String(number=w21, precision (6)=w26) -> (F-format string=w25:string)  [unwired: 2 in]
    n413 = Select(t=w23, s=w22, f=w25) -> (s? t:f=w24:string)
    "Numeric" <- w10
  }
  "MISURE out" <- w8
  "Array" <- w1
